vi "Wait For Plugin Error.vi"(8 "error in (no error)":errorcluster, 9 "timeout in ms (0)":i32 format="%d ms", 11 "Plugin Interface in":refnum<class "Plugin Interface.lvclass">) -> (0 "error out":errorcluster, 2 "error":errorcluster, 3 "Plugin Interface out":refnum<class "Plugin Interface.lvclass">)   [LabVIEW 2017, in "DSF Core.lvlib" / "Plugin Interface.lvclass"]
uses:
  Plugin Interface.lvclass
  C:/Git/DSF/Data Sharing Framework/Source/Core/Engine/Classes/Interfaces/Interface/Interface.lvclass
  Interface/Interface.lvclass/Interface.ctl
  Interface/Read Error Queue.vi
  Dispatcher/Error Timeout.vi
  Interface/Interface.lvclass
  DSF Core.lvlib
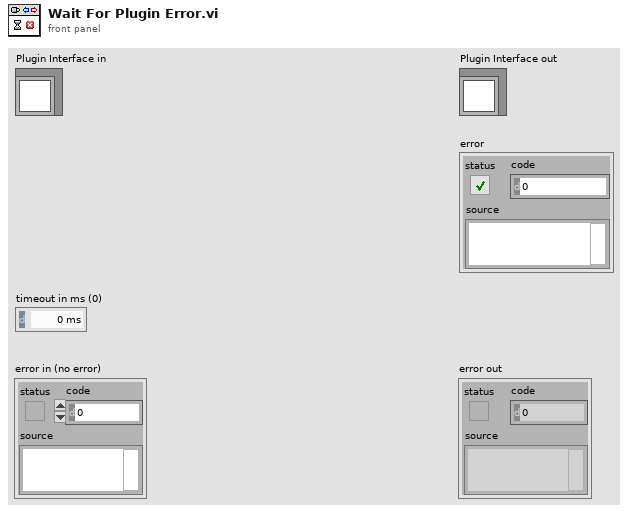
[diagram p1: front panel]
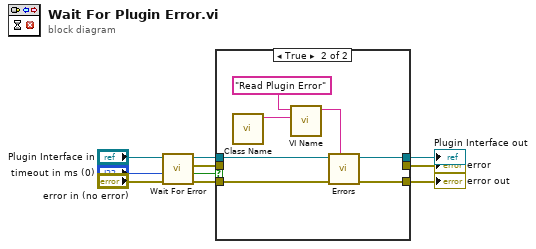
[diagram p0: block diagram]
diagram:
  n1 = call "Wait For Error.vi"("error in (no error)"="error in (no error)", "timeout in ms (0)"="timeout in ms (0)", "Interface in"="Plugin Interface in") -> ("error out"=w6:errorcluster, "timed out?"=w5:bool, "error"=w7:errorcluster, "Interface out"=w4:refnum<class "Plugin Interface.lvclass">)  [unwired: 5 in]
  n2 = case shown="True" w5 {
    tunnel: w6 -> [w12 w19]
    tunnel: w7 -> [w11 _]
    tunnel: w4 -> [w13 w20]
    tunnel: [w13 w18] -> w3
    tunnel: [w12 w17] -> w1
    tunnel: [w11 _] -> w2
    frame False {
    }
    frame True {
      n3 = call "Class Name.vi"() -> ("class name"=w15:string)  [unwired: 11 in]
      n4 = call "VI Name.vi"("class name (\"\")"=w15, "vi name"="Read Plugin Error" ("error source vi name")) -> ("full VI name"=w14:string)  [unwired: 9 in]
      n5 = call-poly "Errors.vi"("error source vi name"=w14, "error in (no error)"=w19, "Interface in"=w20) -> ("error out"=w17:errorcluster, "Interface out"=w18:refnum<class "Plugin Interface.lvclass">)  [unwired: 7 in]
    }
  }
  "error out" <- w1
  "Plugin Interface out" <- w3
  "error" <- w2
